vi "Write RxTx.lvclass.vi"(8 "error in (no error)":errorcluster, 10 "RxTx.lvclass":refnum<class "RxTx.lvclass">, 11 "Communication Channel in":refnum<class "Communication Channel.lvclass">) -> (0 "error out":errorcluster, 3 "Communication Channel out":refnum<class "Communication Channel.lvclass">)   [LabVIEW 2018, in "Communication Channel.lvclass"]
uses:
  Communication Channel.lvclass
  RxTx/RxTx.lvclass
  Communication Channel.lvclass/Communication Channel.ctl
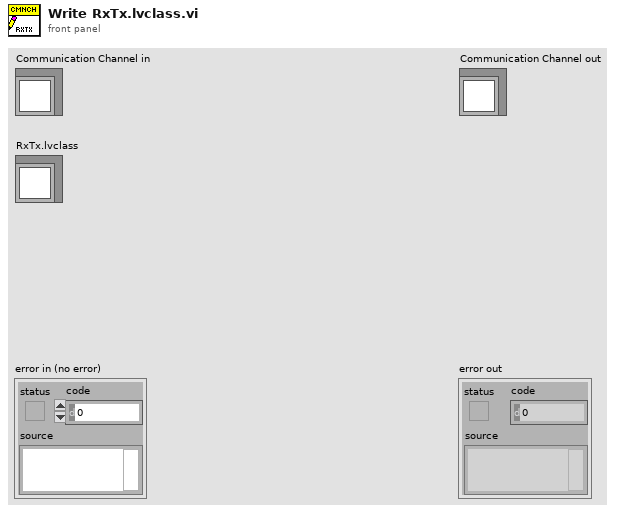
[diagram p1: front panel]
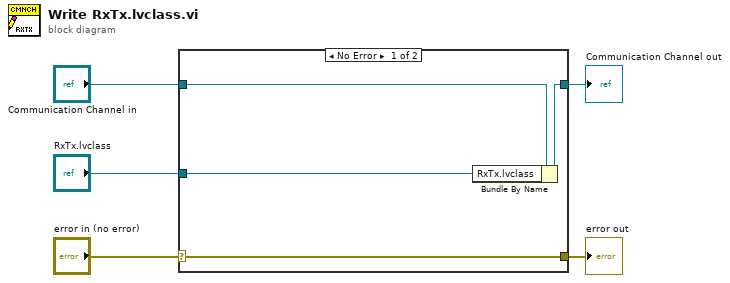
[diagram p0: block diagram]
diagram:
  n1 = case shown="No Error" "error in (no error)" {
    selector: "error in (no error)" -> [w9 w10]
    tunnel: [w9 w10] -> w4
    tunnel: [w7 w11] -> w2
    tunnel: "Communication Channel in" -> [w8 w11]
    tunnel: "RxTx.lvclass" -> [w6 _]
    frame No Error {
      n2 = Bundle By Name(cluster=w8, "RxTx.lvclass"=w6) -> (w7:refnum<class "Communication Channel.lvclass">)
    }
    frame Error {
    }
  }
  "error out" <- w4
  "Communication Channel out" <- w2
